vi "Check Status No Objects - Analog Output.vi"(8 "error in (no error)":errorcluster, 11 "Analog Output in":T1) -> (0 "error out":errorcluster, 1 "Status":string, 2 "Ready?":bool, 3 "Analog Output out":T1)   [LabVIEW 2012]
doc: "(Dynamic) Check if the instrument is powered on and update its member fields with the instrument's current status. Optionally return a text status message."
uses:
  <resource>/objmgr/daqmx.rc
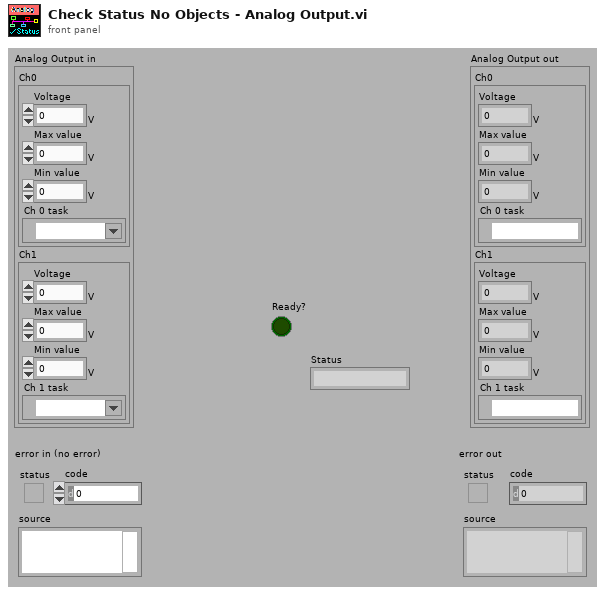
[diagram p1: front panel]
types:
  T1 = cluster{"Ch0":cluster{"Voltage":dbl[unit], "Max value":dbl[unit], "Min value":dbl[unit], "Ch 0 task":refnum<k21>}, "Ch1":cluster{"Voltage":dbl[unit], "Max value":dbl[unit], "Min value":dbl[unit], "Ch 1 task":refnum<k21>}}
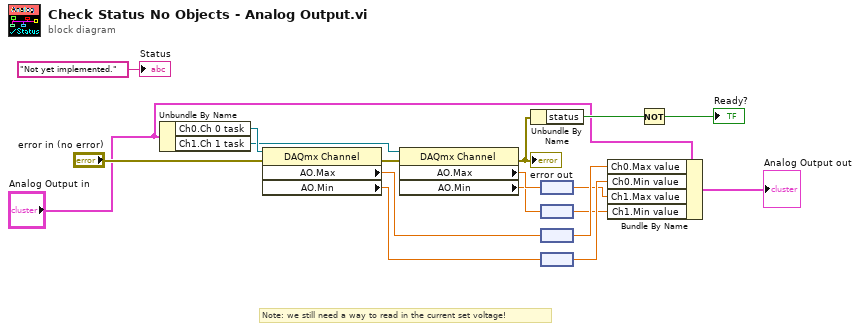
[diagram p0: block diagram]
diagram:
  # "Note: we still need a way to read in the current set voltage!"
  n1 = Unbundle By Name("Analog Output in") -> ("Ch0.Ch 0 task"=w7:refnum<k21>, "Ch1.Ch 1 task"=w6:refnum<k21>)
  n2 = property class="DAQmx Channel"(reference=w7, error in="error in (no error)") -> (error out=w5:errorcluster, "AO.Max"=w18:dbl, "AO.Min"=w16:dbl)  [unwired: 1 out]
  n3 = property class="DAQmx Channel"(reference=w6, error in=w5) -> (error out=w4:errorcluster, "AO.Max"=w14:dbl, "AO.Min"=w12:dbl)  [unwired: 1 out]
  "error out" <- w4
  n4 = Unbundle By Name(w4) -> ("status"=w10:bool)
  n5 = node(w14) -> (w13:dbl[unit])
  n6 = node(w12) -> (w11:dbl[unit])
  n7 = node(w18) -> (w17:dbl[unit])
  n8 = node(w16) -> (w15:dbl[unit])
  n9 = Bundle By Name(cluster="Analog Output in", "Ch0.Max value"=w17, "Ch0.Min value"=w15, "Ch1.Max value"=w13, "Ch1.Min value"=w11) -> (→"Analog Output out":T1)
  n10 = Not(x=w10) -> (.not. x?=→"Ready?":bool)
  "Status" <- "Not yet implemented." ("Status")
